vi "expand tree item.vi"(7 "defer fp updates?(T)":bool=TRUE, 8 "error in (no error)":errorcluster, 9 "Tag":string, 11 "Application Data in":T1) -> (0 "error out":errorcluster, 1 "item children":string[](array[string]), 3 "Application Data out":T1)   [LabVIEW 2017]
uses:
  Application Data.ctl
  DSF Configuration API/1.0.0/Public/Controls/DSF Config Data RefNum.ctl
  Window State.ctl
  DSF Configuration API/1.0.0/Public/Read Item/Read Plugin.vi
  DSF Configuration API/1.0.0/Public/Read Item/Read Group.vi
  DSF Configuration API/1.0.0/Public/Read Item/Read Transfer.vi
  DSF Configuration API/1.0.0/DSF Configuration API.lvlib
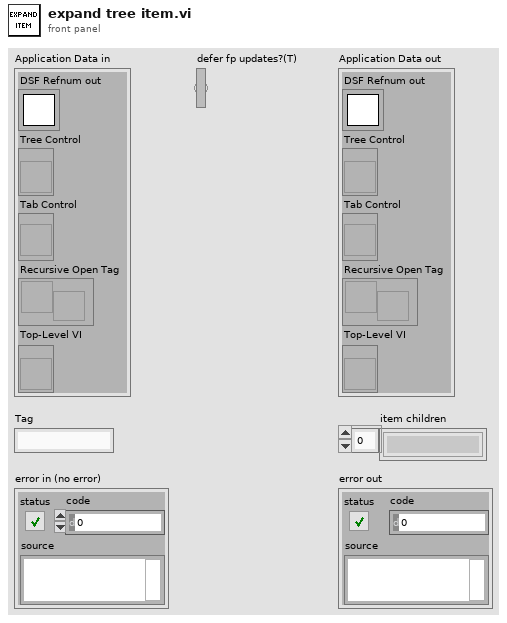
[diagram p1: front panel]
types:
  T1 = typedef "Application Data.ctl" = cluster{"DSF Refnum out":T2, "Tree Control":refnum<vi>, "Tab Control":refnum<vi>, "Recursive Open Tag":refnum<user-event>, "Top-Level VI":refnum<vi>}
  T2 = typedef "DSF Configuration API.lvlib/DSF Config Data RefNum.ctl" = refnum<k1>
  T3 = typedef "Tree Item Type.ctl" = enum16{"Plugin", "Group", "Transfer", "Channel", "Setting"}
  T4 = typedef "DSF Configuration API.lvlib/DSF Plugin Info.ctl" = cluster{"type":string, "timing":T5, "group ids":string[], "settings id":string}
  T5 = typedef "DSF Configuration API.lvlib/DSF Timing Info.ctl" = cluster{"decimation":i32, "offset":i32}
  T6 = cluster{"Left Cell String":string, "Child Text":string[], "Child Tag":string, "Item Indent":i32, "Child Only?":bool, "Glyph Index":i32}[]
  T7 = typedef "DSF Configuration API.lvlib/DSF Group Info.ctl" = cluster{"direction":i32, "timing":T5, "transfer ids":string[], "settings id":string}
  T8 = typedef "DSF Configuration API.lvlib/DSF Transfer Info.ctl" = cluster{"byte order":i32, "channel ids":string[], "settings id":string}
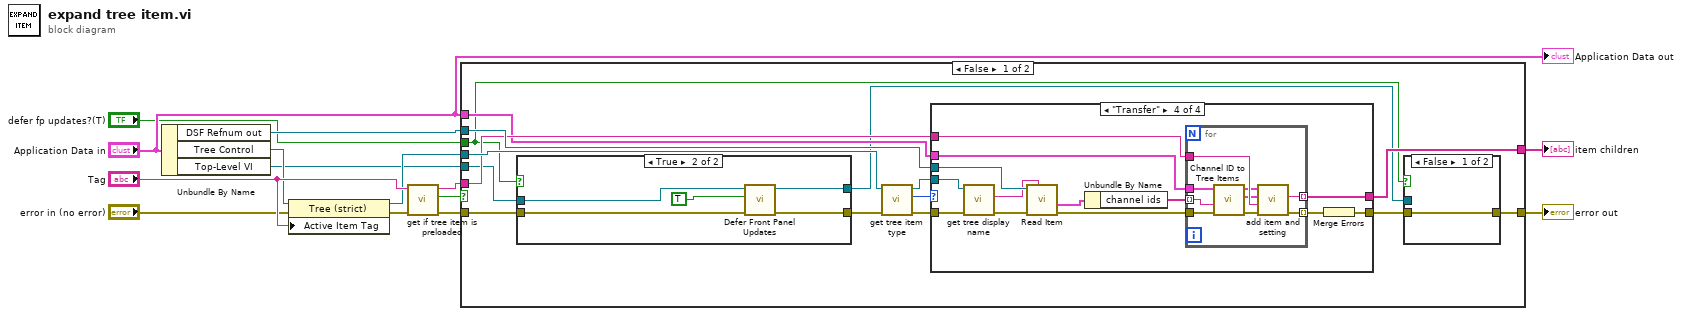
[diagram p0: block diagram]
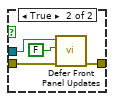
[diagram p2: hidden frame]
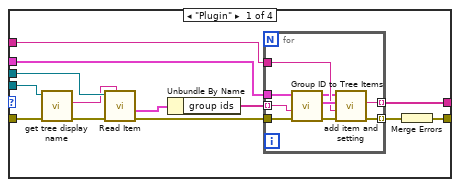
[diagram p4: hidden frame]
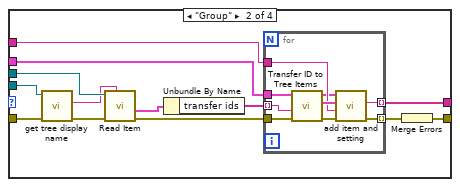
[diagram p5: hidden frame]
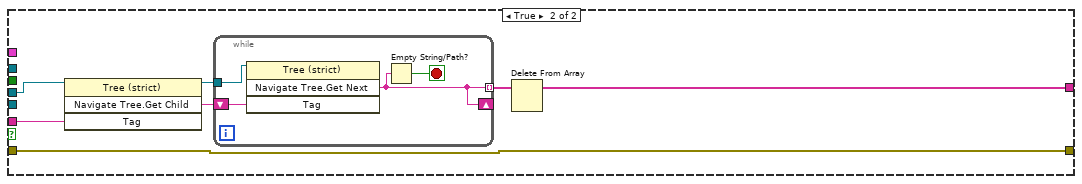
[diagram p7: hidden frame]
diagram:
  n1 = Unbundle By Name("Application Data in") -> ("DSF Refnum out"=w5:T2, "Tree Control"=w4:refnum<vi>, "Top-Level VI"=w2:refnum<vi>)
  n2 = property class="Tree (strict)"(reference=w4, error in="error in (no error)", "Active Item Tag"="Tag") -> (reference out=w8:refnum<vi>, error out=w10:errorcluster)
  n3 = call "get if tree item is preloaded.vi"("error in (no error)"=w10, "Tag in"="Tag") -> ("error out"=w11:errorcluster, "replaced"=w13:bool, "Tag out"=w14:string)  [unwired: 7 in]
  n4 = case shown="False" w13 {
    tunnel: w5 -> [w28 _]
    tunnel: w8 -> [w25 w113]
    tunnel: [w17 w114] -> w9
    tunnel: w11 -> [w24 w114]
    tunnel: w14 -> [w23 w112]
    tunnel: [w22 w109] -> w6
    tunnel: "Application Data in" -> [w20 _]
    tunnel: w2 -> [w19 _]
    tunnel: "defer fp updates?(T)" -> [w15 _]
    frame False {
      n5 = case shown="True" w15 {
        tunnel: w24 -> [w35 w40]
        tunnel: w19 -> [_ w39]
        tunnel: [w35 w37] -> w18
        tunnel: [_ w36] -> w16
        frame False {
        }
        frame True {
          n6 = call "Defer Front Panel Updates.vi"("error in (no error)"=w40, "Defer Panel Updates"=TRUE, "VI in"=w39) -> ("error out"=w37:errorcluster, "VI out"=w36:refnum<vi>)  [unwired: 7 in]
        }
      }
      n7 = call "get tree item type.vi"("error in (no error)"=w18, "TreeControl in"=w25) -> ("error out"=w29:errorcluster, "Item Type"=w27:T3, "TreeControl out"=w21:refnum<vi>)  [unwired: 7 in]
      n8 = case shown="\"Transfer\"" w27 {
        tunnel: w21 -> [w53 w75 _ w98]
        tunnel: w29 -> [w52 w74 w85 w97]
        tunnel: w28 -> [w51 w73 _ w96]
        tunnel: [w45 w67 w85 w91] -> w26
        tunnel: w23 -> [w43 w65 _ w89]
        tunnel: [w42 w64 _ w87] -> w22
        tunnel: w20 -> [w41 w63 _ w86]
        frame "Plugin" {
          n9 = call "get tree display name.vi"("error in (no error)"=w52, "TreeControl in"=w53) -> ("error out"=w50:errorcluster, "display name"=w44:string)  [unwired: 7 in, 1 out]
          n10 = call-poly "Read Item.vi"("name"=w44, "error in (no error)"=w50, "refnum"=w51) -> ("error out"=w47:errorcluster, "value"=w49:T4)  [unwired: 5 in, 2 out]
          n11 = Unbundle By Name(w49) -> ("group ids"=w48:string[])
          n12 = for {
            tunnel: w48 -> [w62] mode=indexing
            tunnel: w47 -> [w61]
            tunnel: [w59] -> w46 mode=indexing
            tunnel: w43 -> [w57]
            tunnel: [w56] -> w42 mode=indexing
            tunnel: w41 -> [w55]
            n13 = call "Group ID to Tree Items.vi"("error in (no error)"=w61, "Group ID"=w62, "Application Data in"=w55) -> ("error out"=w60:errorcluster, "Items"=w58:T6, "Application Data out"=w54:T1)  [unwired: 6 in]
            n14 = call "add item and setting.vi"("error in (no error)"=w60, "Tag"=w57, "items"=w58, "Application Data in"=w54) -> ("error out"=w59:errorcluster, "new item tag"=w56:string)  [unwired: 5 in, 1 out]
          }
          n15 = Merge Errors(w46) -> (w45:errorcluster)
        }
        frame "Group" {
          n16 = call "get tree display name.vi"("error in (no error)"=w74, "TreeControl in"=w75) -> ("error out"=w72:errorcluster, "display name"=w68:string)  [unwired: 7 in, 1 out]
          n17 = call-poly "Read Item.vi"("name"=w68, "error in (no error)"=w72, "refnum"=w73) -> ("error out"=w69:errorcluster, "value"=w71:T7)  [unwired: 5 in, 2 out]
          n18 = Unbundle By Name(w71) -> ("transfer ids"=w70:string[])
          n19 = for {
            tunnel: w70 -> [w84] mode=indexing
            tunnel: w69 -> [w83]
            tunnel: [w81] -> w66 mode=indexing
            tunnel: w65 -> [w79]
            tunnel: [w78] -> w64 mode=indexing
            tunnel: w63 -> [w76]
            n20 = call "Transfer ID to Tree Items.vi"("error in (no error)"=w83, "Transfer ID"=w84, "Application Data in"=w76) -> ("error out"=w82:errorcluster, "tree items"=w80:T6, "Application Data out"=w77:T1)  [unwired: 6 in]
            n21 = call "add item and setting.vi"("error in (no error)"=w82, "Tag"=w79, "items"=w80, "Application Data in"=w77) -> ("error out"=w81:errorcluster, "new item tag"=w78:string)  [unwired: 5 in, 1 out]
          }
          n22 = Merge Errors(w66) -> (w67:errorcluster)
        }
        frame "Channel", "Setting" {
        }
        frame "Transfer" {
          n23 = call "get tree display name.vi"("error in (no error)"=w97, "TreeControl in"=w98) -> ("error out"=w95:errorcluster, "display name"=w92:string)  [unwired: 7 in, 1 out]
          n24 = call-poly "Read Item.vi"("name"=w92, "error in (no error)"=w95, "refnum"=w96) -> ("error out"=w93:errorcluster, "value"=w94:T8)  [unwired: 5 in, 2 out]
          n25 = Unbundle By Name(w94) -> ("channel ids"=w88:string[])
          n26 = for {
            tunnel: w88 -> [w107] mode=indexing
            tunnel: w93 -> [w106]
            tunnel: [w102] -> w90 mode=indexing
            tunnel: w89 -> [w105]
            tunnel: [w101] -> w87 mode=indexing
            tunnel: w86 -> [w100]
            n27 = call "Channel ID to Tree Items.vi"("error in (no error)"=w106, "Channel ID"=w107, "Application Data in"=w100) -> ("error out"=w103:errorcluster, "items"=w104:T6, "Application Data out"=w99:T1)  [unwired: 6 in]
            n28 = call "add item and setting.vi"("error in (no error)"=w103, "Tag"=w105, "items"=w104, "Application Data in"=w99) -> ("error out"=w102:errorcluster, "new item tag"=w101:string)  [unwired: 5 in, 1 out]
          }
          n29 = Merge Errors(w90) -> (w91:errorcluster)
        }
      }
      n30 = case shown="False" w15 {
        tunnel: w26 -> [w30 w34]
        tunnel: [w30 w33] -> w17
        tunnel: w16 -> [_ w32]
        frame False {
        }
        frame True {
          n31 = call "Defer Front Panel Updates.vi"("error in (no error)"=w34, "Defer Panel Updates"=FALSE, "VI in"=w32) -> ("error out"=w33:errorcluster)  [unwired: 7 in, 1 out]
        }
      }
    }
    frame True {
      n32 = invoke class="Tree (strict)" method="Navigate Tree.Get Child"(reference=w113, "Tag"=w112) -> (reference out=w111:refnum<vi>, "Navigate Tree:Get Child"=w108:string)  [unwired: 2 in, 2 out]
      n33 = while {
        tunnel: w111 -> [w118]
        tunnel: [w115] -> w110 mode=indexing
        shift-right: [w115] -> _
        shift-left: w108 -> [w116]
        stop <- w117 stop-if-true
        n34 = invoke class="Tree (strict)" method="Navigate Tree.Get Next"(reference=w118, "Tag"=w116) -> ("Navigate Tree:Get Next Item"=w115:string)  [unwired: 2 in, 3 out]
        n35 = Empty String/Path?(string/path=w115) -> (empty?=w117:bool)
      }
      n36 = Delete From Array(array=w110) -> (array with subset deleted=w109:string[])  [unwired: 2 in, 1 out]
    }
  }
  "error out" <- w9
  "item children" <- w6
  "Application Data out" <- "Application Data in"
